vi "Remove Trailing 0s.vi"(10 "Array":dbl[](array[numeric])) -> (2 "Removed Trail":dbl[](array[numeric]))   [LabVIEW 2014, in "Melody Extraction.lvlib"]
uses:
  Melody Extraction.lvlib
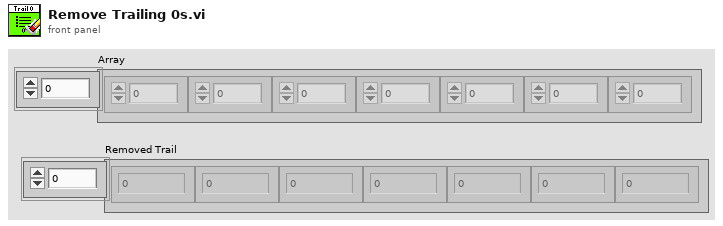
[diagram p1: front panel]
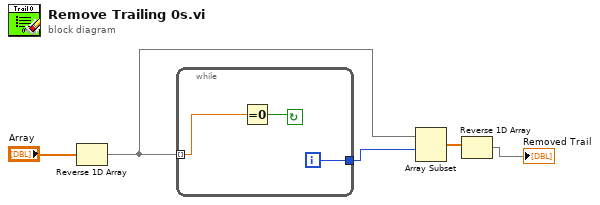
[diagram p0: block diagram]
diagram:
  n1 = Reverse 1D Array(array="Array") -> (reversed array=w4:dbl[])
  n2 = while {
    tunnel: w4 -> [w7] mode=indexing
    tunnel: [w6] -> w3
    i -> [w6]
    stop <- w8 continue-if-true
    n3 = Equal To 0?(x=w7) -> (x = 0?=w8:bool)
  }
  n4 = Array Subset(array=w4, index=w3) -> (w2:dbl[])  [unwired: 1 in]
  n5 = Reverse 1D Array(array=w2) -> (reversed array=→"Removed Trail":dbl[])
